vi "PECT - Scan_time gate_counter -XSeries.vi"() -> ()   [LabVIEW 2018]
uses:
  <vilib>/DAQmx/read.llb/DAQmx Read (Counter U32 1Chan 1Samp).vi
  <vilib>/DAQmx/read.llb/DAQmx Read (Analog 2D DBL NChan NSamp).vi
  <vilib>/Instr/_visa.llb/VISA Configure Serial Port (Instr).vi
  <vilib>/DAQmx/create/channels.llb/DAQmx Create Channel (CI-Count Edges).vi
  <vilib>/DAQmx/create/channels.llb/DAQmx Create Channel (AI-Voltage-Basic).vi
  <vilib>/DAQmx/configure/timing.llb/DAQmx Timing (Sample Clock).vi
  <vilib>/DAQmx/configure/trigger.llb/DAQmx Start Trigger (Digital Edge).vi
  <vilib>/DAQmx/miscellaneous.llb/DAQmx Fill In Error Info.vi
  <resource>/objmgr/daqmx.rc
  <vilib>/Platform/NI_3dgraph.lvlib
panel:
  in  "Tab Control 3":enum32{"Control", "Data Processing"}(tab)
  in  "Backdata online":bool caption="Scan"
  in  "Offset":bool
  in  "Open csv":bool
  in  "Scan":bool
  in  "Save Scan mode":bool caption="Save Process"
  in  "Gate 1":dbl=3.0
  in  "Gate 2":dbl=25.0
  in  "Stop Scan":bool
  in  "Right":bool
  in  "Left":bool
  in  "Front":bool
  in  "Back":bool
  in  "Home X":bool
  in  "Home Y":bool
  in  "Stop 3":bool
  in  "Emergency Stop":bool
  in  "Move Distance":dbl=5.0
  in  "Open tdms":bool
  in  "Pulse frequency":dbl=1000.0 format="%0.2p"
  in  "Pulser Cycles":i32=10
  in  "Sensor No.":i32
  in  "Graph":bool
  in  "Sensor Index":dbl[](array[numeric])=[5.0, 10.0, 12.0, 15.0, 19.0]
  in  "Inverse":bool caption="Scan"
  in  "Trim data":bool caption="Scan"
  in  "X-min":dbl
  in  "X-max":dbl
  in  "Y-min":dbl
  in  "Y-max":dbl
  in  "ViewMode":i32(ring) items=["cwViewXYPlane", "cwViewXZPlane", "cwViewYZPlane", "cwViewUserDefined"]
  in  "Plot style":i32(ring)=5 items=["cwLine"=1, "cwPoint"=2, "cwLinePoint"=3, "cwHiddenLine"=4, "cwSurface"=5, "cwSurfaceLine"=6, "cwSurfaceNormal"=7, "cwContourLine"=8, "cwSurfaceContour"=9]
  in  "Repair Line Col":bool
  in  "Repair Line Row":bool
  in  "Line Col":dbl=167.0
  in  "Line Row":dbl
  in  "low cutoff freq":dbl=40.0 format="%0.2f"
  in  "Filter":bool caption="Scan"
  in  "Backdata":bool caption="Scan"
  in  "Odd":bool caption="Scan"
  in  "DiffY":bool caption="Scan"
  in  "DiffX":bool caption="Scan"
  in  "ColorMapAutoScale":bool=TRUE
  in  "Max":dbl=0.6
  in  "Min":dbl=-0.8
  in  "Abs":bool caption="Scan"
  in  "Backindex":i32
  out "Completed":bool
  out "Start Pos. X":dbl=-55.0 format="%#.4f"
  out "Start. Pos.Y":dbl=-76.83 format="%#.4f"
  in  "Tab Control 2":T1(tab)
  out "Hall sensors signal":dbl[][](graph)
  out "Feature Extraction":dbl(graph)
  in  "3D Surface":refnum<k7>(container)
  out "Record path":path caption="selected path"
  out "Feature extraction scan":dbl[](graph)
  in  "Tab Control":T2(tab)=enum."          DAQ        "
  in  "Step X":dbl=0.5
  out "Move X":bool
  in  "Direction (+)":bool=TRUE
  in  "Step Y":dbl=1.0
  in  "Y-length":dbl=1.0
  in  "X-length":dbl=30.0
  in  "Save Speed":bool
  in  "Cur. Pos Y":dbl=18.8 format="%#.4f"
  in  "Cur. Pos X":dbl=-22.5 format="%#.4f"
  in  "Travel per Pulse (mm)":dbl=0.002
  in  "2 Rate":dbl=0.2
  in  "1 Rate":dbl=0.2
  in  "2 Min":dbl=1.0
  in  "1  Max":dbl=8.0
  in  "2 Max":dbl=8.0
  in  "1 Min":dbl=1.0
  in  "Parity":u16(ring) items=["None", "Odd", "Even", "Mark", "Space"]
  in  "stop bits":u16(ring)=10 items=["1.0"=10, "1.5"=15, "2.0"=20]
  in  "Data bits":u16=8 min=5 max=8 step=1
  in  "Baud Rate":u32=9600
  in  "COM Port":refnum<visa-resource-name>="COM3"
  out "No. X":i32
  out "No. Y":i32
  in  "Counter Terminal":tag="/Dev3/PFI8"
  in  "Counter source":tag="Dev3/ctr0"
  out "No. Data":i32
  out "Motor Pulse Count":u32
  in  "Edge":i32(ring)=10280 items=["Rising"=10280, "Falling"=10171]
  in  "Pulser edge terminal":tag="/Dev3/PFI0"
  out "Sample per Channel AI":dbl
  out "Actual Sample Rate":dbl=500000.0 format="%0.2f"
  in  "Physical Channel":tag="Dev3/ai0:31"
  in  "Min Voltage":dbl=-10.0
  in  "Max Voltage":dbl=10.0
  in  "Terminal Configuration":i32(ring)=10083 items=["default"=-1, "RSE"=10083, "NRSE"=10078, "Differential"=10106, "Pseudodifferential"=12529]
  in  "Sample Rate":dbl=30000.0
  in  "Save Scan mode 2":bool caption="Save Process"
  # "Pulse setting"
  # "Data Processing"
  # "Time gate = %T/2"
  # "Motor control"
  # "Color map"
  # "Process"
  # "Repair line"
  # "Hall Sensors Signal"
  # "Feature Extraction"
  # "COM  Setting"
  # "Speed  Setting"
  # "Scan  Setting"
  # "Pulser"
  # "Motor Trigger"
  # "Sensor  Channel"
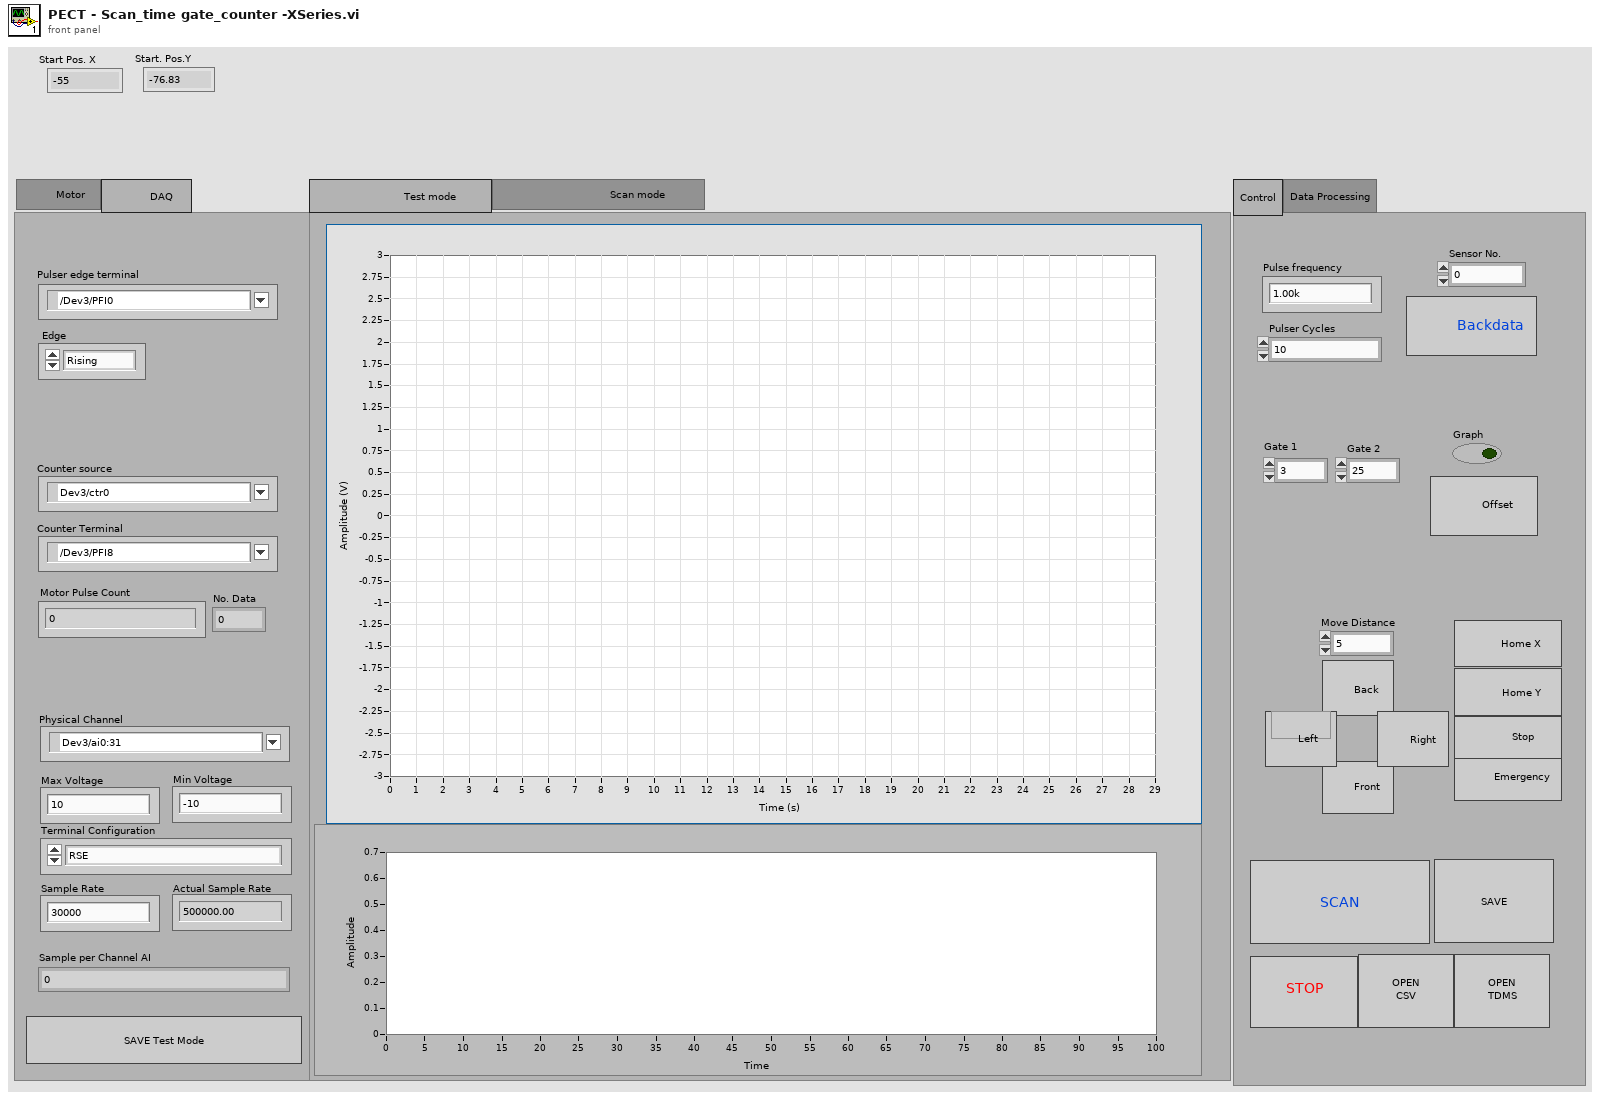
[diagram p1: front panel]
types:
  T1 = enum32{"                    Test mode                   ", "                          Scan mode                      "}
  T2 = enum32{"        Motor      ", "          DAQ        "}
  T3 = enum16{"No Scan", "Move X", "Wait to destination X", "Move Y", "Wait to destinatioin Y"}
  T4 = enum16{"open", "open or create", "create or replace", "create", "open (read-only)"}
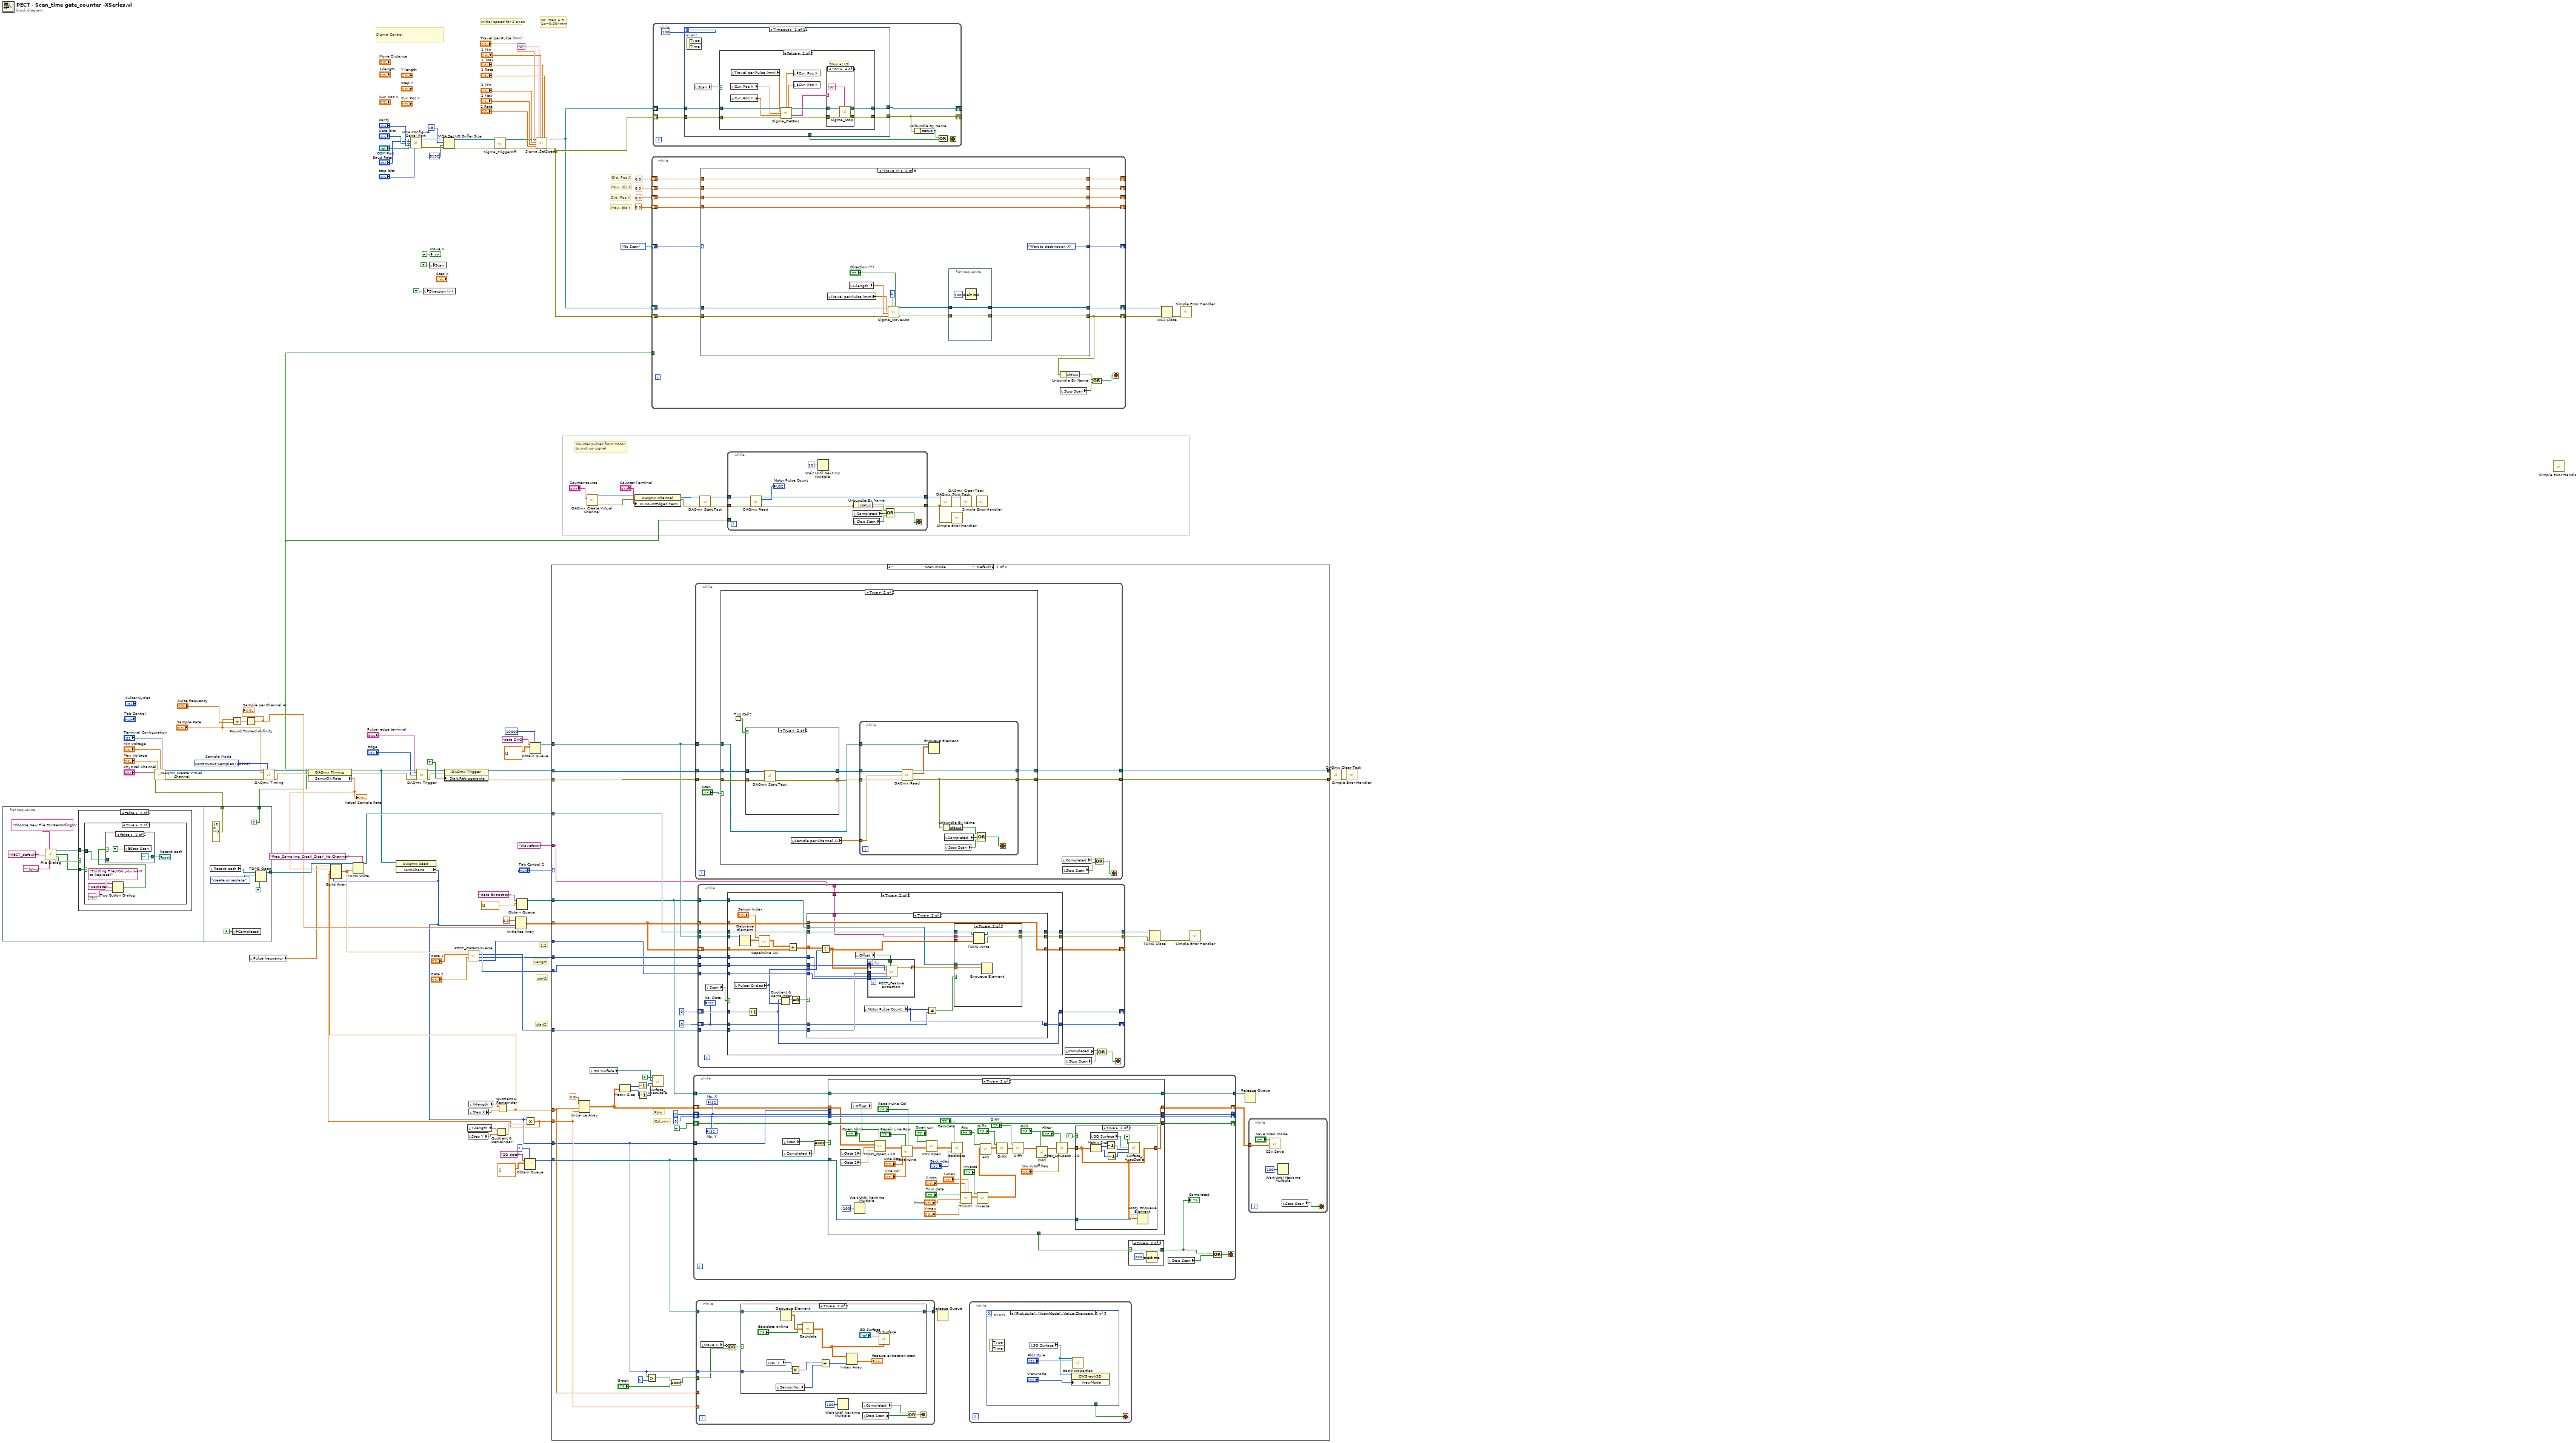
[diagram p0: block diagram]
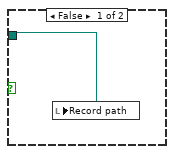
[diagram p2: hidden frame]
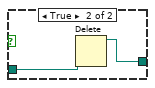
[diagram p3: hidden frame]
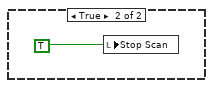
[diagram p4: hidden frame]
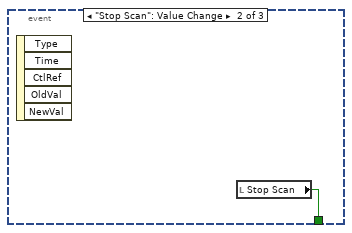
[diagram p5: hidden frame]
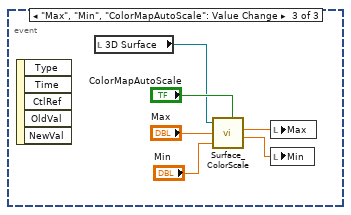
[diagram p6: hidden frame]
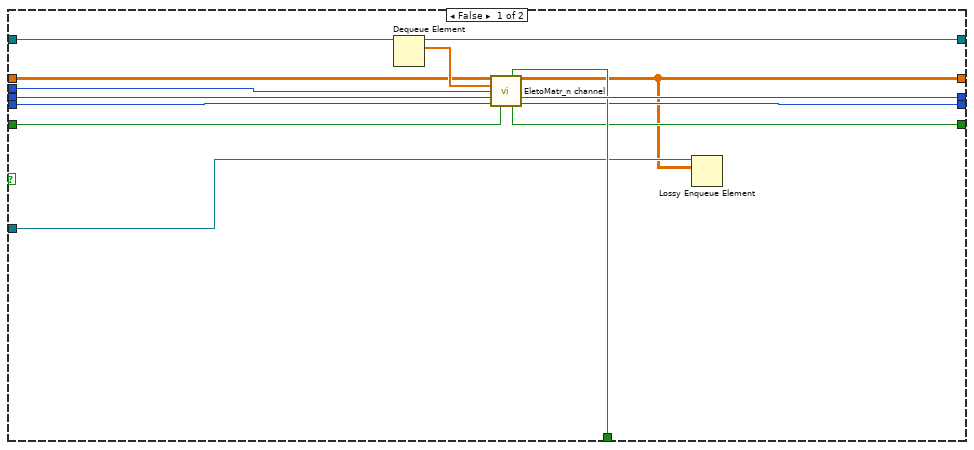
[diagram p9: hidden frame]
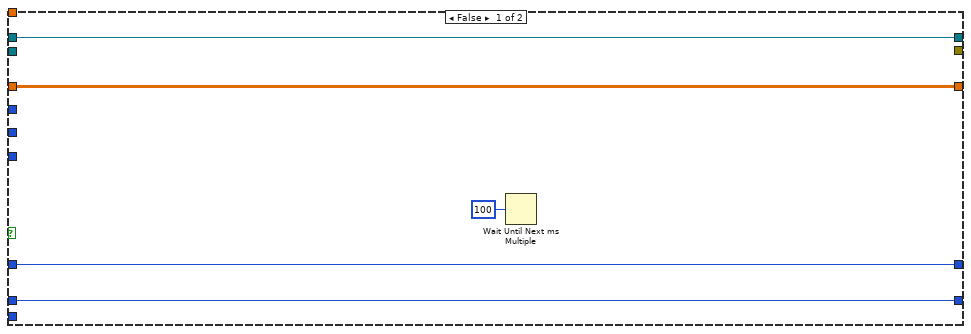
[diagram p13: hidden frame]
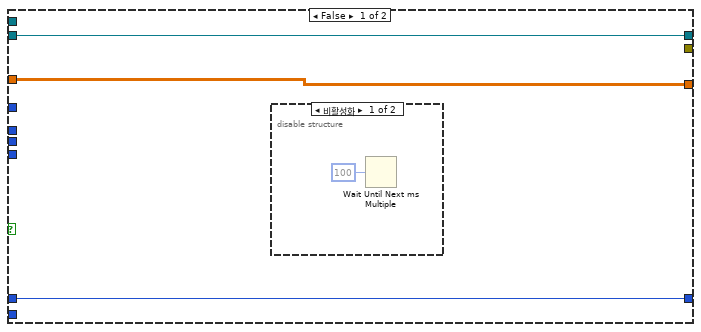
[diagram p14: hidden frame]
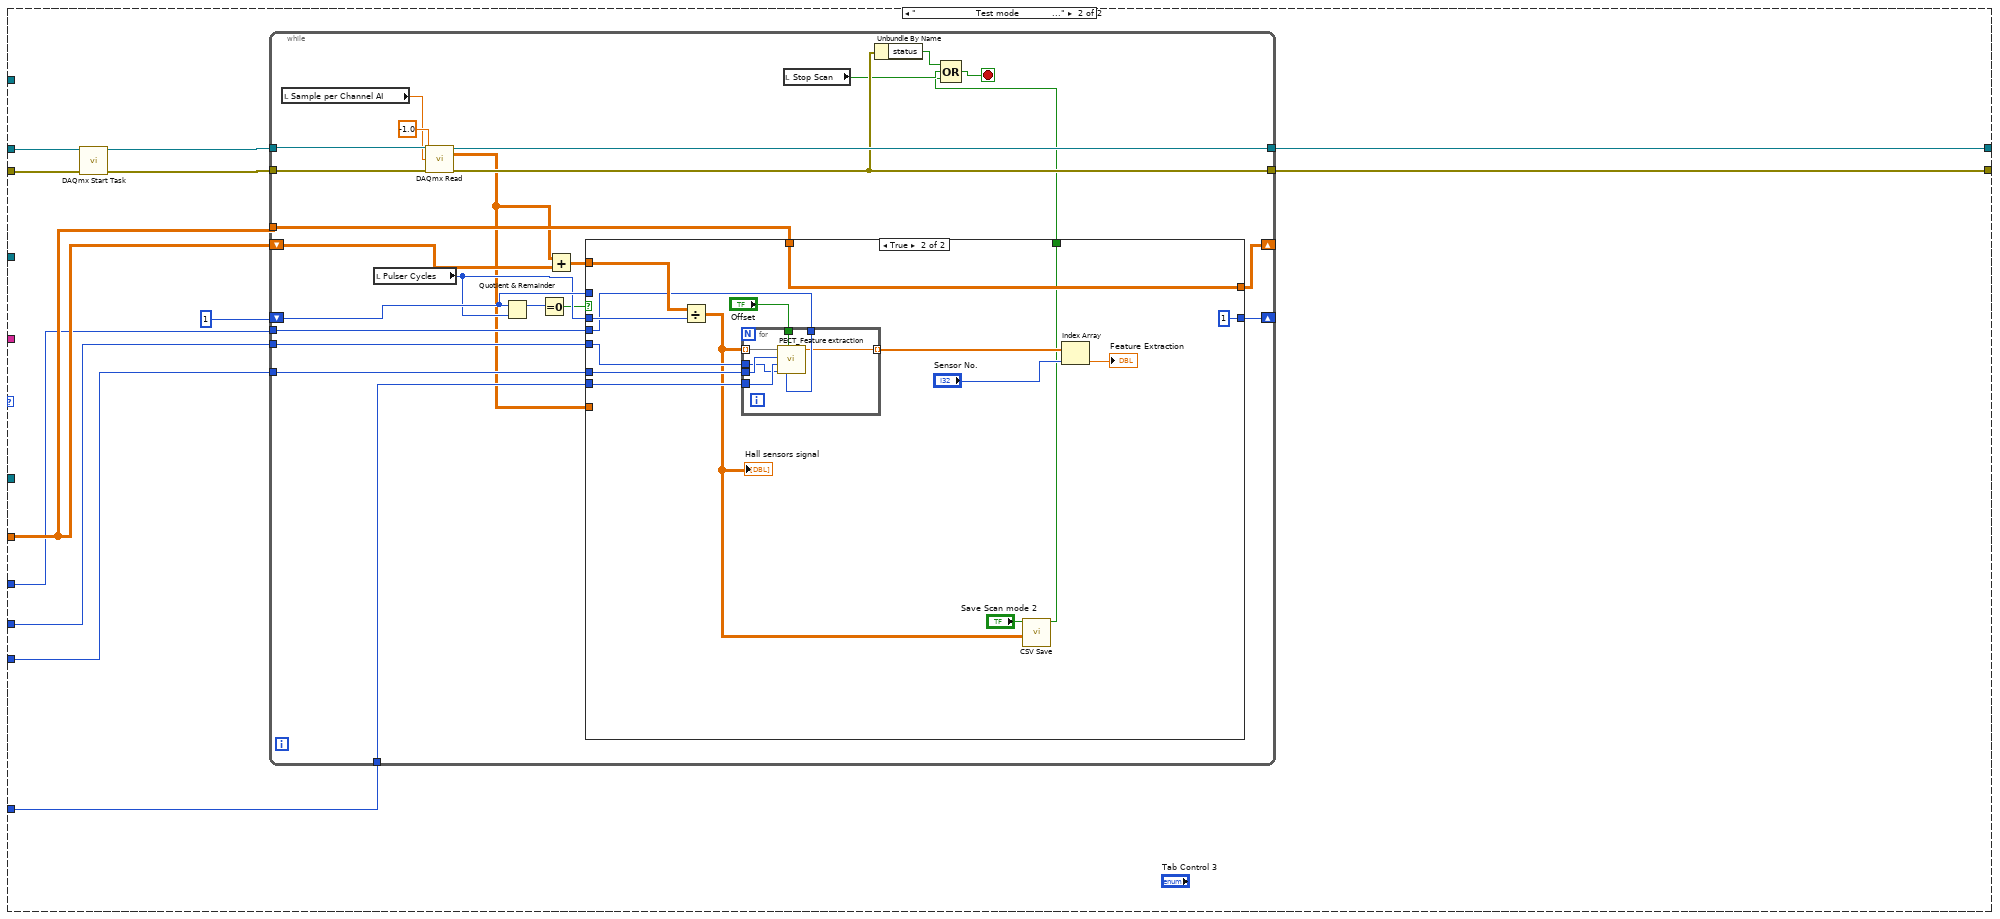
[diagram p17: hidden frame]
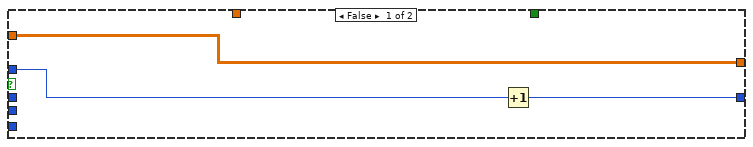
[diagram p18: hidden frame]
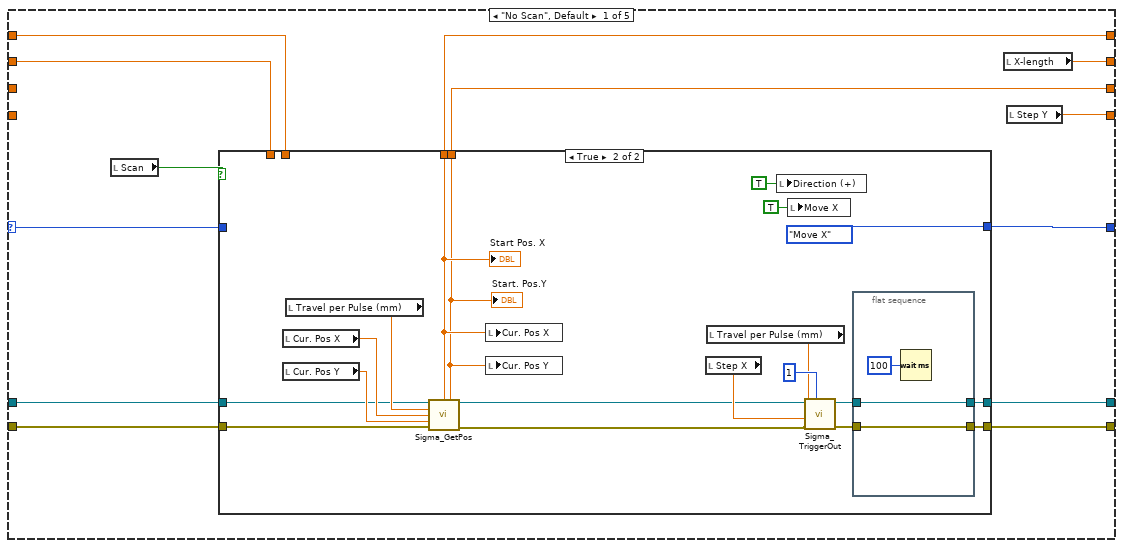
[diagram p19: hidden frame]
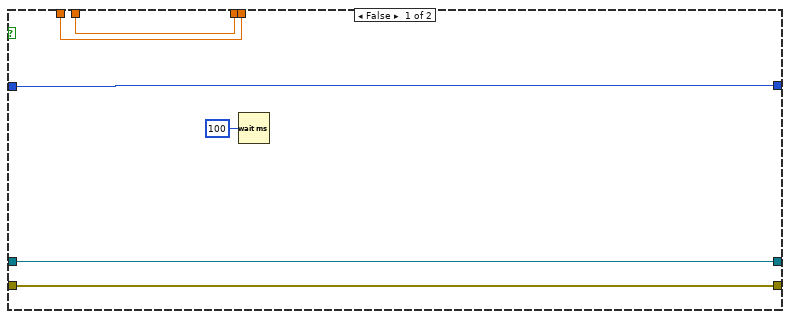
[diagram p20: hidden frame]
diagram:
  w72 = 10123 items=["Finite Samples"=10178, "Continuous Samples"=10123, "Hardware Timed Single Point"=12522]  # Sample Mode
  # "Counter pulses from Motor\nto pick up signal"
  # "1/2"
  # "start1"
  # "start2"
  # "Length"
  # "Mov. dis Y"
  # "Old. Pos Y"
  # "Mov. dis X"
  # "Old. Pos X"
  # "No. step = 5\n1p~0.004mm"
  # "Initial speed for 2 axes"
  # "Sigma Control"
  n1 = flat-sequence {
    tunnel: [w134] -> w57
    tunnel: [TRUE ("disable buffering (T)")] -> w10
    tunnel: [errorcluster {"status"=FALSE, "code"=0, "source"=""} ("error out")] -> w27
    frame #0 {
      n2 = call "File Dialog"("prompt"="Choose New File For Recording\n" ("button label"), "default name"="PECT_default", "pattern (all files)"="*.tdms") -> ("selected path"=w115:path, "exists"=w110:bool, "cancelled"=w111:bool)  [unwired: 9 in, 1 out]
      n3 = case shown="False" w111 {
        tunnel: w115 -> [w116 _]
        tunnel: w110 -> [w117 _]
        frame False {
          n4 = case shown="True" w117 {
            tunnel: w116 -> [w118 w119]
            frame False {
              n5 = local write "Record path"(w118) -> ()
            }
            frame True {
              n6 = Two Button Dialog(message="Existing File\nDo you want to Replace?", 1:"No" ("F button name (\"Cancel\")"), 2:"Replace" ("T button name (\"OK\")")) -> (T button?=w120:bool)
              n7 = case shown="False" w120 {
                tunnel: w119 -> [_ w128]
                tunnel: [path "" ("deleted path") w127] -> w121
                frame False {
                  n8 = local write "Stop Scan"(TRUE ("Exit")) -> ()
                }
                frame True {
                  n9 = Delete(path (use dialog)=w128) -> (deleted path=w127:path)  [unwired: 4 in, 2 out]
                }
              }
              "Record path" <- w121
            }
          }
        }
        frame True {
          n10 = local write "Stop Scan"(TRUE ("Exit")) -> ()
        }
      }
    }
    frame #1 {
      n11 = local read "Record path"() -> (w133:path)
      n12 = local write "Completed"(FALSE ("Completed")) -> ()
      n13 = TDMS Open(6:FALSE ("disable buffering (T)"), 10:T4."create or replace" ("operation"), 11:w133) -> (3:w134:refnum<k34>)  [unwired: 4 in, 1 out]
    }
  }
  n14 = call-poly <vilib>:"DAQmx Create Virtual Channel.vi"("maximum value"="Max Voltage", "minimum value"="Min Voltage", "input terminal configuration"="Terminal Configuration", "physical channels"="Physical Channel", "error in"=w27) -> ("task out"=w81:refnum<k21>, "error out"=w82:errorcluster)  [unwired: 9 in]
  n15 = Divide(x="Sample Rate", y="Pulse frequency") -> (x/y=w59:dbl)
  n16 = Round Toward -Infinity(1:w59) -> (0:w32:dbl)
  "Sample per Channel AI" <- w32
  n17 = local read "Pulse frequency"() -> (w30:dbl)
  n18 = call-poly <vilib>:"DAQmx Timing.vi"("task/channels in"=w81, "sample mode"=w72, "rate"="Sample Rate", "error in"=w82) -> ("task out"=w33:refnum<k21>, "error out"=w83:errorcluster)  [unwired: 10 in]
  n19 = property class="DAQmx Timing"(reference=w33, error in=w83) -> (reference out=w6:refnum<k21>, error out=w3:errorcluster, "SampClk.Rate"=w35:dbl)
  "Actual Sample Rate" <- w35
  n20 = property class="DAQmx Read"(reference=w6) -> ("NumChans"=w26:u32)  [unwired: 1 in, 2 out]
  n21 = call-poly "VISA Configure Serial Port"("VISA resource name"="COM Port", "baud rate (9600)"="Baud Rate", "data bits (8)"="Data bits", "parity (0:none)"="Parity", "stop bits (10: 1 bit)"="stop bits") -> ("VISA resource name out"=w96:refnum<visa-resource-name>, "error out"=w102:errorcluster)  [unwired: 9 in]
  n22 = call-poly <vilib>:"DAQmx Trigger.vi"("task/channels in"=w6, "source"="Pulser edge terminal", "edge"="Edge", "error in"=w3) -> ("task out"=w8:refnum<k21>, "error out"=w7:errorcluster)  [unwired: 10 out]
  n23 = local write "Direction (+)"(TRUE ("Scan")) -> ()
  n24 = local write "Scan"(FALSE ("Scan")) -> ()
  n25 = VISA Set I/O Buffer Size(VISA resource name=w96, mask (16)=48, size (4096)=u32 8192, error in (no error)=w102) -> (VISA resource name out=w44:refnum<visa-resource-name>, error out=w43:errorcluster)
  n26 = property class="DAQmx Trigger"(reference=w8, error in=w7, "Start.Retriggerable"=TRUE) -> (reference out=w5:refnum<k21>, error out=w4:errorcluster)
  n27 = local read "Y-length"() -> (w61:dbl)
  n28 = local read "Step Y"() -> (w62:dbl)
  n29 = local read "X-length"() -> (w64:dbl)
  n30 = local read "Step X"() -> (w63:dbl)
  n31 = call "Sigma_TriggerOff.vi"("error in (no error)"=w43, "VISA resource name"=w44) -> ("error out"=w41:errorcluster, "VISA resource name out"=w42:refnum<visa-resource-name>)  [unwired: 8 in]
  n32 = Quotient & Remainder(x=w61, y=w62) -> (floor(x/y)=w28:dbl)  [unwired: 1 out]
  n33 = Quotient & Remainder(x=w64, y=w63) -> (floor(x/y)=w55:dbl)  [unwired: 1 out]
  n34 = Initialize Array(0.0 ("element"), w26, w32) -> (w69:dbl[][])
  n35 = Obtain Queue(name (unnamed)="data Extraction", element data type=dbl[] [] ("data")) -> (queue out=w66:refnum<queue>)  [unwired: 3 in, 2 out]
  n36 = Obtain Queue(max queue size (-1, unlimited)=2 ("최대 큐 크기(-1,제한없음)"), name (unnamed)="2D data", element data type=dbl[][] [] ("initialized array")) -> (queue out=w37:refnum<queue>)  [unwired: 2 in, 2 out]
  n37 = Multiply(x=w26, y=w28) -> (x*y=w25:dbl)
  n38 = Build Array(w30, w35, w55, w25, w26) -> (w40:dbl[])
  n39 = TDMS Write(0:w57, 5:"Freq_Sampling_SizeX_SizeY_No.Channel" ("group name in (Untitled)"), 9:w40) -> (4:w56:refnum<k34>)  [unwired: 3 in, 3 out]
  n40 = call "PECT_GateConverse.vi"("Gate 2"="Gate 2", "Gate 1"="Gate 1", "Freq_Sampling_SizeX_SizeY"=w40) -> ("Length T/2"=w45:i32, "Length"=w46:i32, "Start 2"=w47:i32, "Start 1"=w48:i32)  [unwired: 4 in, 1 out]
  n41 = Obtain Queue(max queue size (-1, unlimited)=10000, name (unnamed)="data DAQ", element data type=dbl[][] [] ("data")) -> (queue out=w68:refnum<queue>)  [unwired: 2 in, 2 out]
  n42 = call "Sigma_SetSpeed.vi"("VISA resource name"=w42, "Travel per Pulse (0.004mm)"="Travel per Pulse (mm)", "Min (1mm) 2"="2 Min", "Max (2mm) 2"="2 Max", "Rate (1mm) 2"="2 Rate", "error in (no error)"=w41, "Axis (1)"="W", "Min (1mm)"="1 Min", "Max (2mm)"="1  Max", "Rate (1mm)"="1 Rate") -> ("VISA resource name out"=w108:refnum<visa-resource-name>, "error out"=w109:errorcluster)  [unwired: 8 in]
  n43 = case shown="\"                          Scan mode                      \", Default" "Tab Control 2" {
    tunnel: w5 -> [w176 w430]
    tunnel: [w175 w438] -> w75
    tunnel: [w174 w437] -> w74
    tunnel: w69 -> [w171 w436]
    tunnel: w4 -> [w173 w429]
    tunnel: w45 -> [w172 w435]
    tunnel: w68 -> [w170 _]
    tunnel: w66 -> [w150 _]
    tunnel: w55 -> [w145 _]
    tunnel: w25 -> [w146 _]
    tunnel: w46 -> [w158 w433]
    tunnel: w48 -> [w157 w432]
    tunnel: w47 -> [w156 w431]
    tunnel: w56 -> [w155 _]
    tunnel: "Waveform" ("group name in (Untitled)") -> [w152 _]
    tunnel: w37 -> [w147 _]
    tunnel: w26 -> [w141 _]
    frame "                          Scan mode                      ", Default {
      # "Column"
      # "Row"
      n44 = Initialize Array(0.0 ("element"), w145, w146) -> (w142:dbl[][])
      n45 = local read "3D Surface"() -> (w159:refnum<k7>)
      n46 = Matrix Size(0:w142) -> (1:w164:i32, 2:w165:i32)
      n47 = Decrement(x=w164) -> (x-1=w168:i32)
      n48 = Decrement(x=w165) -> (x-1=w167:i32)
      n49 = Greater?(x=w141, y=u32 1) -> (0:w139:bool)
      n50 = call "Surface_AxesScale.vi"("Y-axis Max"=w167, "X-axis max"=w168, "3D Surface"=w159, "Auto Scale"=FALSE) -> ()  [unwired: 8 in]
      n51 = Compound Arithmetic op=AND(w139, "Graph") -> (w137:bool)
      n52 = while {
        shift-right: [w231] -> _
        shift-left: 0 -> [w233]
        shift-right: [w230] -> _
        shift-left: 0 -> [w232]
        tunnel: w150 -> [w229]
        shift-right: [w221] -> w143
        shift-left: w142 -> [w228]
        shift-right: [w224] -> _
        shift-left: TRUE ("Output Direction") -> [w225]
        tunnel: w147 -> [w223]
        tunnel: [w222] -> w148
        tunnel: w141 -> [w217]
        stop <- w226 stop-if-true
        n53 = local read "Scan"() -> (w220:bool)
        n54 = local read "Completed"() -> (w219:bool)
        n55 = Compound Arithmetic op=AND(invert w220, invert w219) -> (w218:bool)
        n56 = case shown="True" w218 {
          tunnel: w233 -> [w250 w293]
          tunnel: w232 -> [w249 w292]
          tunnel: [w248 w293] -> w231
          tunnel: [w243 w292] -> w230
          tunnel: w229 -> [w247 w284]
          tunnel: w228 -> [w238 w289]
          tunnel: [w241 w271] -> w221
          tunnel: [w246 _] -> w216
          tunnel: w225 -> [w245 w291]
          tunnel: [w244 w291] -> w224
          tunnel: w223 -> [w242 w273]
          tunnel: [w237 w284] -> w222
          tunnel: w217 -> [w239 _]
          frame False {
            n57 = Dequeue Element(queue=w247) -> (queue out=w237:refnum<queue>, element=w240:dbl[])  [unwired: 2 in, 2 out]
            n58 = call "EletoMatr_n channel.vi"("Input Array X"=w238, "Input data"=w240, "No. channels"=w239, "In Row"=w250, "In Column"=w249, "Input Direction"=w245) -> ("Completed"=w246:bool, "Out Array X"=w241:dbl[][], "Out Row"=w248:i32, "Output Direction"=w244:bool, "Out Column"=w243:i32)  [unwired: 5 in]
            n59 = Lossy Enqueue Element(queue=w242, element=w241) -> ()  [unwired: 1 in, 4 out]
          }
          frame True {
            n60 = local read "Gate 1"() -> (w288:dbl)
            n61 = local read "Gate 2"() -> (w287:dbl)
            n62 = local read "Offset"() -> (w278:bool)
            n63 = Wait Until Next ms Multiple(millisecond multiple=u32 100 ("ms 배수")) -> ()  [unwired: 1 out]
            n64 = call "TDMS_Open - 1D.vi"("Offset"=w278, "Gate 2"=w287, "Gate 1"=w288, "Input 2D"=w289, "Open"="Open tdms") -> ("Output 2D"=w265:dbl[][])  [unwired: 5 in, 1 out]
            n65 = call "RepairLine.vi"("Repair Line Col"="Repair Line Col", "Repair Line Row"="Repair Line Row", "Line Col"="Line Col", "Line Row"="Line Row", "Array In"=w265) -> ("Array Repaired"=w264:dbl[][])  [unwired: 6 in]
            n66 = call "CSV Open.vi"("2D Array In"=w264, "Open"="Open csv") -> ("2D Array Out"=w272:dbl[][])  [unwired: 9 in]
            n67 = call "Backdata.vi"("Backindex"="Backindex", "Array in"=w272, "Backdata"="Backdata") -> ("Array out"=w259:dbl[][])
            n68 = call "TrimXY.vi"("X-max"="Y-max", "X-min"="Y-min", "Y-max"="X-max", "Y-min"="X-min", "Array In"=w259, "Trim data"="Trim data") -> ("Array Trim Out"=w253:dbl[][])  [unwired: 5 in]
            n69 = call "Inverse.vi"(10:"Inverse"=w253, 11:"Inverse"="Inverse") -> ("Array out"=w251:dbl[][])  [unwired: 9 in]
            n70 = call "Abs.vi"("Input"=w251, "Abs"="Abs") -> ("Array out"=w277:dbl[][])  [unwired: 9 in]
            n71 = call "DiffX.vi"("Array in"=w277, "DiffX"="DiffX") -> ("Array out"=w282:dbl[][])  [unwired: 1 in]
            n72 = call "DiffY.vi"("Array in"=w282, "DiffY"="DiffY") -> ("Array out"=w280:dbl[][])  [unwired: 1 in]
            n73 = call "Odd.vi"("Odd"="Odd", "Array In"=w280) -> ("Array Out"=w269:dbl[][])  [unwired: 9 in]
            n74 = call "Filter_Lowpass - 2D.vi"("Filter"="Filter", "Input 2D"=w269, "low cutoff freq: fl"="low cutoff freq") -> ("Output"=w268:dbl[][])  [unwired: 6 in]
            n75 = case shown="True" TRUE {
              tunnel: w268 -> [w294 w295]
              tunnel: [w294 w295] -> w271
              tunnel: w273 -> [_ w296]
              frame False {
              }
              frame True {
                n76 = local read "3D Surface"() -> (w300:refnum<k7>)
                n77 = Matrix Size(0:w295) -> (1:w301:i32, 2:w298:i32)
                n78 = Decrement(x=w301) -> (x-1=w299:i32)
                n79 = Decrement(x=w298) -> (x-1=w297:i32)
                n80 = call "Surface_AxesScale.vi"("Y-axis Max"=w297, "X-axis max"=w299, "3D Surface"=w300, "Auto Scale"=FALSE) -> ()  [unwired: 8 in]
                n81 = Lossy Enqueue Element(queue=w296, element=w295) -> ()  [unwired: 1 in, 4 out]
              }
            }
          }
        }
        n82 = case shown="True" w216 {
          selector: w216 -> [w234 w235]
          tunnel: [w234 w235] -> w215
          frame False {
          }
          frame True {
            n83 = Wait (ms)(milliseconds to wait=u32 200) -> ()  [unwired: 1 out]
          }
        }
        "Completed" <- w215
        n84 = local read "Stop Scan"() -> (w227:bool)
        n85 = Compound Arithmetic op=OR(w215, w227) -> (w226:bool)
        "No. Y" <- w232
        "No. X" <- w233
      }
      n86 = while {
        tunnel: w176 -> [w311]
        tunnel: [w310] -> w175
        tunnel: [w309] -> w174
        tunnel: w173 -> [w308]
        tunnel: w170 -> [w307]
        stop <- w303 stop-if-true
        n87 = case shown="True" "Scan" {
          tunnel: w311 -> [w313 w320]
          tunnel: [w313 w322] -> w310
          tunnel: [w312 w321] -> w309
          tunnel: w308 -> [w312 w319]
          tunnel: w307 -> [_ w316]
          frame False {
          }
          frame True {
            n88 = First Call?() -> (First Call?: T/F=w315:bool)
            n89 = case shown="True" w315 {
              tunnel: w320 -> [w324 w328]
              tunnel: w319 -> [w323 w327]
              tunnel: [w324 w326] -> w318
              tunnel: [w323 w325] -> w317
              frame False {
              }
              frame True {
                n90 = call <vilib>:"DAQmx Start Task.vi"("task/channels in"=w328, "error in"=w327) -> ("task out"=w326:refnum<k21>, "error out"=w325:errorcluster)  [unwired: 12 in]
              }
            }
            n91 = local read "Sample per Channel AI"() -> (w314:dbl)
            n92 = while {
              tunnel: [w339] -> w322
              tunnel: [w338] -> w321
              tunnel: w316 -> [w337]
              tunnel: w318 -> [w332]
              tunnel: w317 -> [w331]
              tunnel: w314 -> [w329]
              stop <- w333 stop-if-true
              n93 = call-poly <vilib>:"DAQmx Read.vi"("task/channels in"=w332, "number of samples per channel"=w329, "error in"=w331) -> ("task out"=w339:refnum<k21>, "data"=w330:dbl[][], "error out"=w338:errorcluster)  [unwired: 10 in]
              n94 = Enqueue Element(queue=w337, element=w330) -> ()  [unwired: 2 in, 3 out]
              n95 = Unbundle By Name(w338) -> ("status"=w334:bool)
              n96 = local read "Completed"() -> (w336:bool)
              n97 = local read "Stop Scan"() -> (w335:bool)
              n98 = Compound Arithmetic op=OR(w334, w336, w335) -> (w333:bool)
            }
          }
        }
        n99 = local read "Completed"() -> (w304:bool)
        n100 = local read "Stop Scan"() -> (w305:bool)
        n101 = Compound Arithmetic op=OR(w304, w305) -> (w303:bool)
      }
      n102 = while {
        tunnel: w147 -> [w195]
        tunnel: w146 -> [_]
        tunnel: w145 -> [_]
        tunnel: [w198] -> w144
        tunnel: w141 -> [w197]
        tunnel: w137 -> [w193]
        stop <- w199 stop-if-true
        n103 = local read "Move X"() -> (w194:bool)
        n104 = Compound Arithmetic op=OR(invert w194, w193) -> (w192:bool)
        n105 = case shown="True" w192 {
          tunnel: [w202 w212] -> w198
          tunnel: w197 -> [_ w210]
          tunnel: w195 -> [w202 w206]
          frame False {
          }
          frame True {
            n106 = local read "No. Y"() -> (w211:i32)
            n107 = local read "Sensor No."() -> (w208:i32)
            n108 = Dequeue Element(queue=w206) -> (queue out=w212:refnum<queue>, element=w205:dbl[][])  [unwired: 2 in, 2 out]
            n109 = Multiply(x=w211, y=w210) -> (x*y=w209:u32)
            n110 = call "Backdata.vi"("Array in"=w205, "Backdata"="Backdata online") -> ("Array out"=w204:dbl[][])  [unwired: 1 in]
            n111 = Add(x=w209, y=w208) -> (x+y=w207:u32)
            n112 = Index Array(array=w204, index (col)=w207) -> (element=→"Feature extraction scan":dbl[])  [unwired: 1 in]
            n113 = call <vilib>:"3D Surface.vi"("z matrix"=w204, "3D graph"="3D Surface") -> ()  [unwired: 8 in, 2 out]
          }
        }
        n114 = Wait Until Next ms Multiple(millisecond multiple=u32 100 ("ms 배수")) -> ()  [unwired: 1 out]
        n115 = local read "Completed"() -> (w196:bool)
        n116 = local read "Stop Scan"() -> (w200:bool)
        n117 = Compound Arithmetic op=OR(w196, w200) -> (w199:bool)
      }
      n118 = while {
        shift-right: [w356] -> _
        shift-left: w171 -> [w360]
        tunnel: w171 -> [w359]
        tunnel: w172 -> [w358]
        tunnel: w170 -> [w357]
        tunnel: w150 -> [w355]
        shift-right: [w352] -> _
        shift-left: 0 -> [w353]
        tunnel: w158 -> [w351]
        tunnel: w157 -> [w350]
        tunnel: w156 -> [w349]
        tunnel: w155 -> [w348]
        tunnel: [w347] -> w154
        tunnel: [w346] -> w153
        tunnel: w152 -> [w345]
        shift-right: [w344] -> _
        shift-left: 0 -> [w340]
        stop <- w341 stop-if-true
        n119 = local read "Scan"() -> (w354:bool)
        n120 = case shown="True" w354 {
          tunnel: w360 -> [w365 w381]
          tunnel: w359 -> [_ w386]
          tunnel: w358 -> [_ w385]
          tunnel: w357 -> [_ w384]
          tunnel: [w365 w383] -> w356
          tunnel: w355 -> [_ w382]
          tunnel: w353 -> [w364 w379]
          tunnel: [w364 w378] -> w352
          tunnel: w351 -> [_ w377]
          tunnel: w350 -> [_ w376]
          tunnel: w349 -> [_ w375]
          tunnel: w348 -> [w362 w374]
          tunnel: [w362 w373] -> w347
          tunnel: [_ w372] -> w346
          tunnel: w345 -> [_ w371]
          tunnel: w340 -> [w361 w370]
          tunnel: [w361 w369] -> w344
          frame False {
            n121 = Wait Until Next ms Multiple(millisecond multiple=u32 100 ("ms 배수")) -> ()  [unwired: 1 out]
          }
          frame True {
            n122 = local read "Pulser Cycles"() -> (w380:i32)
            n123 = Dequeue Element(queue=w384) -> (element=w368:dbl[][])  [unwired: 2 in, 3 out]
            n124 = Increment(x=w379) -> (x+1=w378:i32)
            n125 = call "RepairLine 2D.vi"("Array in"=w368, "Sensor Index"="Sensor Index") -> ("Array Out"=w366:dbl[][])  [unwired: 9 in]
            n126 = Quotient & Remainder(x=w378, y=w380) -> (x-y*floor(x/y)=w387:i32)  [unwired: 1 out]
            n127 = Add(x=w366, y=w381) -> (x+y=w389:dbl[][])
            n128 = Equal To 0?(x=w387) -> (x = 0?=w388:bool)
            n129 = case shown="True" w388 {
              tunnel: w380 -> [_ w410]
              tunnel: w389 -> [w392 w408]
              tunnel: [w392 w411] -> w383
              tunnel: w386 -> [_ w411]
              tunnel: w385 -> [_ w404]
              tunnel: w382 -> [_ w409]
              tunnel: w377 -> [_ w405]
              tunnel: w376 -> [_ w407]
              tunnel: w375 -> [_ w406]
              tunnel: w374 -> [w391 w400]
              tunnel: [w391 w397] -> w373
              tunnel: [_ w396] -> w372
              tunnel: w371 -> [_ w399]
              tunnel: w370 -> [w390 w401]
              tunnel: [w390 w395] -> w369
              frame False {
                n130 = disable-structure shown="비활성화" {
                  frame Disabled {
                    n131 = Wait Until Next ms Multiple(millisecond multiple=u32 100 ("ms 배수")) -> ()  [unwired: 1 out]
                  }
                  frame Enabled {
                  }
                }
              }
              frame True {
                n132 = Divide(x=w408, y=w410) -> (x/y=w398:dbl[][])
                n133 = local read "Offset"() -> (w403:bool)
                n134 = local read "Motor Pulse Count"() -> (w395:u32)
                n135 = for {
                  tunnel: w407 -> [w418]
                  tunnel: w406 -> [w417]
                  tunnel: w405 -> [w416]
                  tunnel: w404 -> [w415]
                  tunnel: w403 -> [w414]
                  tunnel: [w413] -> w402 mode=indexing
                  tunnel: w398 -> [w412] mode=indexing
                  n136 = call "PECT_Feature extraction.vi"("Length T/2"=w415, "Offset"=w414, "Length"=w416, "Start 2"=w417, "Start 1"=w418, "Pulse signal in"=w412) -> ("Feature extraction out"=w413:dbl)  [unwired: 5 in]
                }
                n137 = Not Equal?(x=w395, y=w401) -> (x != y?=w394:bool)
                n138 = case shown="True" w394 {
                  tunnel: w409 -> [_ w426]
                  tunnel: w402 -> [_ w425]
                  tunnel: w400 -> [w419 w424]
                  tunnel: w399 -> [_ w423]
                  tunnel: w398 -> [_ w422]
                  tunnel: [w419 w421] -> w397
                  tunnel: [_ w420] -> w396
                  frame False {
                  }
                  frame True {
                    n139 = TDMS Write(0:w424, 5:w423, 9:w422) -> (4:w421:refnum<k34>, 15:w420:errorcluster)  [unwired: 3 in, 2 out]
                    n140 = Enqueue Element(queue=w426, element=w425) -> ()  [unwired: 2 in, 3 out]
                  }
                }
              }
            }
          }
        }
        n141 = local read "Completed"() -> (w343:bool)
        n142 = local read "Stop Scan"() -> (w342:bool)
        n143 = Compound Arithmetic op=OR(w343, w342) -> (w341:bool)
        "No. Data" <- w340
      }
      n144 = Release Queue(queue=w144) -> ()  [unwired: 2 in, 3 out]
      n145 = while {
        stop <- w181 stop-if-true
        n146 = event shown="[0] \"Plot style\", \"ViewMode\": Value Change" {
          selector: _ -> [_ _ _]
          dyn-events: _ -> [_ _ _]
          timeout: _ -> [_ _ _]
          tunnel: [_ w185 _] -> w181
          event "Plot style", "ViewMode": Value Change {
            n147 = event-data() -> ()  [unwired: 1 in, 2 out]
            n148 = local read "3D Surface"() -> (w184:refnum<k7>)
            n149 = property class="CWGraph3D"(reference=w184, "ViewMode"="ViewMode") -> ()  [unwired: 1 in, 2 out]
            n150 = call <vilib>:"Basic Properties.vi"("3D graph"=w184, "plot style"="Plot style") -> ()  [unwired: 12 in, 2 out]
          }
          event "Stop Scan": Value Change {
            n151 = event-data() -> ()  [unwired: 1 in, 5 out]
            n152 = local read "Stop Scan"() -> (w185:bool)
          }
          event "Max", "Min", "ColorMapAutoScale": Value Change {
            n153 = event-data() -> ()  [unwired: 1 in, 5 out]
            n154 = local read "3D Surface"() -> (w186:refnum<k7>)
            n155 = call "Surface_ColorScale.vi"("ColorMapAutoScale"="ColorMapAutoScale", "Min"="Min", "Max"="Max", "3D Surface_"=w186) -> ("Min 2"=w190:dbl, "Max 2"=w189:dbl)  [unwired: 1 in, 2 out]
            n156 = local write "Max"(w189) -> ()
            n157 = local write "Min"(w190) -> ()
          }
        }
      }
      n158 = TDMS Close(8:w153, 11:w154) -> (0:w151:errorcluster)  [unwired: 1 out]
      n159 = call <vilib>:"Simple Error Handler.vi"("error in (no error)"=w151) -> ()  [unwired: 2 in, 7 out]
      n160 = Release Queue(queue=w148) -> ()  [unwired: 2 in, 3 out]
      n161 = while {
        tunnel: w143 -> [w179]
        stop <- w178 stop-if-true
        n162 = call "CSV Save.vi"("Array"=w179, "Save Button"="Save Scan mode") -> ()  [unwired: 9 in, 1 out]
        n163 = Wait Until Next ms Multiple(millisecond multiple=u32 100 ("ms 배수")) -> ()  [unwired: 1 out]
        n164 = local read "Stop Scan"() -> (w178:bool)
      }
    }
    frame "                    Test mode                   " {
      n165 = call <vilib>:"DAQmx Start Task.vi"("task/channels in"=w430, "error in"=w429) -> ("task out"=w428:refnum<k21>, "error out"=w427:errorcluster)  [unwired: 12 in]
      n166 = while {
        tunnel: w428 -> [w446]
        tunnel: w427 -> [w445]
        tunnel: [w461] -> w437
        tunnel: [w462] -> w438
        shift-right: [w458] -> _
        shift-left: w436 -> [w459]
        tunnel: w436 -> [w457]
        tunnel: w435 -> [w455]
        shift-right: [w453] -> _
        shift-left: 1 ("Average") -> [w452]
        tunnel: w433 -> [w450]
        tunnel: w432 -> [w449]
        tunnel: w431 -> [w448]
        stop <- w439 stop-if-true
        n167 = local read "Sample per Channel AI"() -> (w444:dbl)
        n168 = local read "Pulser Cycles"() -> (w451:i32)
        n169 = call-poly <vilib>:"DAQmx Read.vi"("task/channels in"=w446, "number of samples per channel"=w444, "timeout"=-1.0, "error in"=w445) -> ("task out"=w462:refnum<k21>, "data"=w443:dbl[][], "error out"=w461:errorcluster)  [unwired: 9 in]
        n170 = Quotient & Remainder(x=w452, y=w451) -> (x-y*floor(x/y)=w460:i32)  [unwired: 1 out]
        n171 = Equal To 0?(x=w460) -> (x = 0?=w447:bool)
        n172 = Add(x=w443, y=w459) -> (x+y=w456:dbl[][])
        n173 = case shown="True" w447 {
          tunnel: w451 -> [_ w478]
          tunnel: w443 -> [_ _]
          tunnel: w456 -> [w465 w480]
          tunnel: [w465 w479] -> w458
          tunnel: w457 -> [_ w479]
          tunnel: w455 -> [_ w472]
          tunnel: [w463 1 ("Average")] -> w453
          tunnel: w452 -> [w464 _]
          tunnel: w450 -> [_ w474]
          tunnel: w449 -> [_ w476]
          tunnel: w448 -> [_ w475]
          tunnel: [_ w466] -> w440
          frame False {
            n174 = Increment(x=w464) -> (x+1=w463:i32)
          }
          frame True {
            n175 = Divide(x=w480, y=w478) -> (x/y=w467:dbl[][])
            "Hall sensors signal" <- w467
            n176 = for {
              tunnel: w467 -> [w487] mode=indexing
              tunnel: w476 -> [w486]
              tunnel: w475 -> [w485]
              tunnel: w474 -> [w484]
              tunnel: "Offset" -> [w483]
              tunnel: w472 -> [w482]
              tunnel: [w481] -> w471 mode=indexing
              n177 = call "PECT_Feature extraction.vi"("Length T/2"=w482, "Offset"=w483, "Length"=w484, "Start 2"=w485, "Start 1"=w486, "Pulse signal in"=w487) -> ("Feature extraction out"=w481:dbl)  [unwired: 5 in]
            }
            n178 = call "CSV Save.vi"("Array"=w467, "Save Button"="Save Scan mode 2") -> ("Save Status"=w466:bool)  [unwired: 9 in]
            n179 = Index Array(array=w471, index="Sensor No.") -> (element=→"Feature Extraction":dbl)
          }
        }
        n180 = local read "Stop Scan"() -> (w441:bool)
        n181 = Unbundle By Name(w461) -> ("status"=w442:bool)
        n182 = Compound Arithmetic op=OR(w442, w441, w440) -> (w439:bool)
      }
    }
  }
  n183 = call-poly <vilib>:"DAQmx Create Virtual Channel.vi"("counter"="Counter source") -> ("task out"=w18:refnum<k21>, "error out"=w20:errorcluster)  [unwired: 13 in]
  n184 = property class="DAQmx Channel"(reference=w18, error in=w20, "CI.CountEdges.Term"="Counter Terminal") -> (reference out=w13:refnum<k21>, error out=w14:errorcluster)
  n185 = while {
    shift-right: [w503] -> _
    shift-left: T3."No Scan" -> [w504]
    shift-right: [w499] -> _
    shift-left: 0.0 ("Current  Position (mm)") -> [w498]
    shift-right: [w497] -> _
    shift-left: 0.0 ("Current  Position (mm)") -> [w496]
    shift-right: [w495] -> _
    shift-left: 0.0 ("Current  Position (mm)") -> [w494]
    shift-right: [w493] -> _
    shift-left: 0.0 ("Current  Position (mm)") -> [w492]
    shift-right: [w500] -> w52
    shift-left: w108 -> [w502]
    shift-right: [w490] -> w53
    shift-left: w109 -> [w501]
    tunnel: w10 -> [_]
    stop <- w488 stop-if-true
    n186 = case shown="\"Move X\"" w504 {
      selector: w504 -> [w515 _ _ _ _]
      tunnel: [w516 T3."Wait to destination X" w580 w597 w653] -> w503
      tunnel: w502 -> [w510 w549 w574 w602 w644]
      tunnel: w501 -> [w509 w548 w573 w601 w643]
      tunnel: [w512 w551 w579 w599 w650] -> w500
      tunnel: [w511 w550 w578 w598 w649] -> w490
      tunnel: [w508 w556 w577 w616 w656] -> w499
      tunnel: w498 -> [w506 w556 w565 w616 w656]
      tunnel: [w514 w555 w582 w615 w655] -> w497
      tunnel: w496 -> [w505 w555 w582 w615 w655]
      tunnel: [w507 w554 w575 w600 w652] -> w495
      tunnel: w494 -> [_ w554 w575 w600 w638]
      tunnel: [w513 w553 w583 w614 w651] -> w493
      tunnel: w492 -> [_ w553 w583 w614 w651]
      frame "No Scan", Default {
        n187 = local read "Scan"() -> (w517:bool)
        n188 = case shown="True" w517 {
          tunnel: [w523 T3."Move X"] -> w516
          tunnel: w515 -> [w523 _]
          tunnel: w510 -> [w522 w529]
          tunnel: w509 -> [w521 w528]
          tunnel: [w522 w534] -> w512
          tunnel: [w521 w533] -> w511
          tunnel: [w520 w525] -> w508
          tunnel: [w519 w524] -> w507
          tunnel: w506 -> [w520 _]
          tunnel: w505 -> [w519 _]
          frame False {
            n189 = Wait (ms)(milliseconds to wait=u32 100) -> ()  [unwired: 1 out]
          }
          frame True {
            n190 = local read "Cur. Pos X"() -> (w531:dbl)
            n191 = local read "Cur. Pos Y"() -> (w532:dbl)
            n192 = local read "Travel per Pulse (mm)"() -> (w530:dbl)
            n193 = call "Sigma_GetPos.vi"("VISA resource name"=w529, "Travel per Pulse (mm)"=w530, "Init Pos X (mm)"=w531, "Init  Pos Y (mm)"=w532, "error in (no error)"=w528) -> ("Pos X (mm)"=w525:dbl, "Pos Y (mm)"=w524:dbl, "VISA resource name out"=w527:refnum<visa-resource-name>, "error out"=w526:errorcluster)  [unwired: 6 in, 1 out]
            "Start Pos. X" <- w525
            "Start. Pos.Y" <- w524
            n194 = local write "Cur. Pos X"(w525) -> ()
            n195 = local write "Cur. Pos Y"(w524) -> ()
            n196 = local read "Step X"() -> (w538:dbl)
            n197 = local read "Travel per Pulse (mm)"() -> (w537:dbl)
            n198 = local write "Direction (+)"(TRUE ("Direction (+)")) -> ()
            n199 = local write "Move X"(TRUE ("Move X")) -> ()
            n200 = call "Sigma_TriggerOut.vi"("Axis(1)"=1, "error in (no error)"=w526, "Trigger distance (mm)"=w538, "Travel per Pulse (mm)"=w537, "VISA resource name"=w527) -> ("error out"=w535:errorcluster, "VISA resource name out"=w536:refnum<visa-resource-name>)  [unwired: 5 in]
            n201 = flat-sequence {
              tunnel: [w545] -> w534
              tunnel: w536 -> [w545]
              tunnel: [w544] -> w533
              tunnel: w535 -> [w544]
              frame #0 {
                n202 = Wait (ms)(milliseconds to wait=u32 100) -> ()  [unwired: 1 out]
              }
            }
          }
        }
        n203 = local read "X-length"() -> (w514:dbl)
        n204 = local read "Step Y"() -> (w513:dbl)
      }
      frame "Move X" {
        n205 = local read "Travel per Pulse (mm)"() -> (w558:dbl)
        n206 = local read "X-length"() -> (w559:dbl)
        n207 = call "Sigma_MoveAbs.vi"("Direction (+)"="Direction (+)", "Axis (1)"=1, "error in (no error)"=w548, "Travel (1mm)"=w559, "Travel per Pulse (0.004mm)"=w558, "VISA resource name"=w549) -> ("error out"=w546:errorcluster, "VISA resource name out"=w547:refnum<visa-resource-name>)  [unwired: 4 in]
        n208 = flat-sequence {
          tunnel: [w563] -> w551
          tunnel: w547 -> [w563]
          tunnel: [w562] -> w550
          tunnel: w546 -> [w562]
          frame #0 {
            n209 = Wait (ms)(milliseconds to wait=u32 100) -> ()  [unwired: 1 out]
          }
        }
      }
      frame "Wait to destination X" {
        n210 = local read "Cur. Pos X"() -> (w570:dbl)
        n211 = local read "Cur. Pos Y"() -> (w569:dbl)
        n212 = local read "Travel per Pulse (mm)"() -> (w576:dbl)
        n213 = call "Sigma_GetPos.vi"("VISA resource name"=w574, "Travel per Pulse (mm)"=w576, "Init Pos X (mm)"=w570, "Init  Pos Y (mm)"=w569, "error in (no error)"=w573) -> ("Pos X (mm)"=w564:dbl, "Pos Y (mm)"=w568:dbl, "VISA resource name out"=w572:refnum<visa-resource-name>, "error out"=w571:errorcluster)  [unwired: 6 in, 1 out]
        n214 = Absolute Value(x=w582) -> (abs(x)=w584:dbl)
        n215 = local write "Cur. Pos X"(w564) -> ()
        n216 = local write "Cur. Pos Y"(w568) -> ()
        n217 = Subtract(x=w564, y=w565) -> (x-y=w586:dbl)
        n218 = Absolute Value(x=w586) -> (abs(x)=w585:dbl)
        n219 = Subtract(x=w585, y=w584) -> (x-y=w567:dbl)
        n220 = call "Convert Double Precision.vi"("Input"=w567) -> ("Output"=w566:dbl)  [unwired: 10 in]
        n221 = Greater Or Equal To 0?(x=w566) -> (x >= 0?=w581:bool)
        n222 = case shown="True" w581 {
          tunnel: [T3."Wait to destination X" T3."Move Y"] -> w580
          tunnel: w572 -> [w589 w593]
          tunnel: w571 -> [w588 w592]
          tunnel: [w589 w593] -> w579
          tunnel: [w588 w592] -> w578
          tunnel: [w587 w594] -> w577
          tunnel: w565 -> [w587 _]
          frame False {
            n223 = disable-structure shown="비활성화" {
              frame Disabled {
                n224 = Wait (ms)(milliseconds to wait=u32 100) -> ()  [unwired: 1 out]
              }
              frame Enabled {
              }
            }
          }
          frame True {
            n225 = local read "Cur. Pos X"() -> (w594:dbl)
            n226 = local write "Move X"(FALSE ("Move X")) -> ()
          }
        }
      }
      frame "Move Y" {
        n227 = local read "Y-length"() -> (w605:dbl)
        n228 = local read "Step Y"() -> (w603:dbl)
        n229 = local read "Start. Pos.Y"() -> (w608:dbl)
        n230 = Subtract(x=w605, y=w603) -> (x-y=w604:dbl)
        n231 = Subtract(x=w608, y=w600) -> (x-y=w613:dbl)
        n232 = Absolute Value(x=w604) -> (abs(x)=w611:dbl)
        n233 = Absolute Value(x=w613) -> (abs(x)=w612:dbl)
        n234 = Subtract(x=w612, y=w611) -> (x-y=w606:dbl)
        n235 = local write "Move X"(FALSE ("Move X")) -> ()
        n236 = call "Convert Double Precision.vi"("Input"=w606) -> ("Output"=w607:dbl)  [unwired: 10 in]
        n237 = Greater Or Equal To 0?(x=w607) -> (x >= 0?=w609:bool)
        n238 = case shown="False" w609 {
          tunnel: [w619 w635] -> w599
          tunnel: [w618 w634] -> w598
          tunnel: w602 -> [w621 w633]
          tunnel: w601 -> [w620 w632]
          tunnel: [T3."Wait to destinatioin Y" T3."No Scan"] -> w597
          frame False {
            n239 = local read "Travel per Pulse (mm)"() -> (w625:dbl)
            n240 = local read "Step Y"() -> (w626:dbl)
            n241 = call "Sigma_MoveAbs.vi"("Direction (+)"=TRUE, "Axis (1)"=2, "error in (no error)"=w620, "Travel (1mm)"=w626, "Travel per Pulse (0.004mm)"=w625, "VISA resource name"=w621) -> ("error out"=w623:errorcluster, "VISA resource name out"=w624:refnum<visa-resource-name>)  [unwired: 4 in]
            n242 = flat-sequence {
              tunnel: [w630] -> w619
              tunnel: w624 -> [w630]
              tunnel: [w629] -> w618
              tunnel: w623 -> [w629]
              frame #0 {
                n243 = Wait (ms)(milliseconds to wait=u32 100) -> ()  [unwired: 1 out]
              }
            }
          }
          frame True {
            n244 = call "Sigma_TriggerOff.vi"("error in (no error)"=w632, "VISA resource name"=w633) -> ("error out"=w634:errorcluster, "VISA resource name out"=w635:refnum<visa-resource-name>)  [unwired: 8 in]
            n245 = local write "Scan"(FALSE ("Move X")) -> ()
          }
        }
      }
      frame "Wait to destinatioin Y" {
        n246 = local read "Cur. Pos X"() -> (w647:dbl)
        n247 = local read "Cur. Pos Y"() -> (w646:dbl)
        n248 = local read "Travel per Pulse (mm)"() -> (w648:dbl)
        n249 = call "Sigma_GetPos.vi"("VISA resource name"=w644, "Travel per Pulse (mm)"=w648, "Init Pos X (mm)"=w647, "Init  Pos Y (mm)"=w646, "error in (no error)"=w643) -> ("Pos X (mm)"=w645:dbl, "Pos Y (mm)"=w637:dbl, "VISA resource name out"=w642:refnum<visa-resource-name>, "error out"=w641:errorcluster)  [unwired: 6 in, 1 out]
        n250 = Absolute Value(x=w651) -> (abs(x)=w657:dbl)
        n251 = Subtract(x=w637, y=w638) -> (x-y=w659:dbl)
        n252 = local write "Cur. Pos X"(w645) -> ()
        n253 = local write "Cur. Pos Y"(w637) -> ()
        n254 = Absolute Value(x=w659) -> (abs(x)=w658:dbl)
        n255 = Subtract(x=w658, y=w657) -> (x-y=w640:dbl)
        n256 = call "Convert Double Precision.vi"("Input"=w640) -> ("Output"=w639:dbl)  [unwired: 10 in]
        n257 = Greater Or Equal To 0?(x=w639) -> (x >= 0?=w654:bool)
        n258 = case shown="False" w654 {
          tunnel: [T3."Wait to destinatioin Y" T3."Move X"] -> w653
          tunnel: w638 -> [w662 _]
          tunnel: [w662 w669] -> w652
          tunnel: [w661 w668] -> w650
          tunnel: [w660 w667] -> w649
          tunnel: w642 -> [w661 w668]
          tunnel: w641 -> [w660 w667]
          frame False {
            n259 = disable-structure shown="비활성화" {
              frame Disabled {
                n260 = Wait (ms)(milliseconds to wait=u32 100) -> ()  [unwired: 1 out]
              }
              frame Enabled {
              }
            }
          }
          frame True {
            n261 = local read "Cur. Pos Y"() -> (w669:dbl)
            n262 = local read "Direction (+)"() -> (w666:bool)
            n263 = local write "Move X"(TRUE ("Move X")) -> ()
            n264 = Not(x=w666) -> (.not. x?=w665:bool)
            n265 = local write "Direction (+)"(w665) -> ()
          }
        }
      }
    }
    n266 = Unbundle By Name(w490) -> ("status"=w489:bool)
    n267 = local read "Stop Scan"() -> (w491:bool)
    n268 = Compound Arithmetic op=OR(w489, w491) -> (w488:bool)
  }
  n269 = while {
    shift-right: [w674] -> _
    shift-left: w108 -> [w679]
    shift-right: [w676] -> _
    shift-left: w109 -> [w678]
    stop <- w675 stop-if-true
    n270 = event shown="[0] Timeout" {
      selector: _ -> [_ _ _ _ _ _ _ _ _ _ _]
      dyn-events: _ -> [_ _ _ _ _ _ _ _ _ _ _]
      timeout: 100 -> [_ _ _ _ _ _ _ _ _ _ _]
      tunnel: w679 -> [w684 w717 w730 w733 w748 w763 w778 w795 w807 w817 w829]
      tunnel: w678 -> [w683 w716 w727 w732 w747 w762 w777 w794 w806 w816 w828]
      tunnel: [w682 w717 w729 w735 w750 w765 w780 w792 w805 w819 w831] -> w674
      tunnel: [w681 w716 w728 w734 w749 w764 w779 w791 w804 w818 w830] -> w676
      tunnel: [_ "Stop Scan" _ _ _ _ _ _ _ _ _] -> w673
      event Timeout {
        n271 = event-data() -> ()  [unwired: 1 in, 2 out]
        n272 = local read "Scan"() -> (w680:bool)
        n273 = case shown="False" w680 {
          tunnel: w684 -> [w696 w715]
          tunnel: w683 -> [w695 w714]
          tunnel: [w694 w715] -> w682
          tunnel: [w693 w714] -> w681
          frame False {
            # "Stop at LS"
            n274 = local read "Cur. Pos X"() -> (w686:dbl)
            n275 = local read "Cur. Pos Y"() -> (w685:dbl)
            n276 = local read "Travel per Pulse (mm)"() -> (w688:dbl)
            n277 = call "Sigma_GetPos.vi"("VISA resource name"=w696, "Travel per Pulse (mm)"=w688, "Init Pos X (mm)"=w686, "Init  Pos Y (mm)"=w685, "error in (no error)"=w695) -> ("Pos X (mm)"=w691:dbl, "Pos Y (mm)"=w692:dbl, "VISA resource name out"=w689:refnum<visa-resource-name>, "State String"=w687:string, "error out"=w690:errorcluster)  [unwired: 6 in]
            n278 = local write "Cur. Pos X"(w691) -> ()
            n279 = local write "Cur. Pos Y"(w692) -> ()
            n280 = case shown="\"W\"" w687 {
              tunnel: [w698 w703 w708 w713] -> w694
              tunnel: [w697 w702 w707 w712] -> w693
              tunnel: w689 -> [w698 w700 w705 w710]
              tunnel: w690 -> [w697 w699 w704 w709]
              frame "K", Default {
              }
              frame "L" {
                n281 = call "Sigma_Stop.vi"("Axis (1)"="1", "error in (no error)"=w699, "VISA resource name"=w700) -> ("error out"=w702:errorcluster, "VISA resource name out"=w703:refnum<visa-resource-name>)  [unwired: 7 in]
              }
              frame "M" {
                n282 = call "Sigma_Stop.vi"("Axis (1)"="2", "error in (no error)"=w704, "VISA resource name"=w705) -> ("error out"=w707:errorcluster, "VISA resource name out"=w708:refnum<visa-resource-name>)  [unwired: 7 in]
              }
              frame "W" {
                n283 = call "Sigma_Stop.vi"("Axis (1)"="W", "error in (no error)"=w709, "VISA resource name"=w710) -> ("error out"=w712:errorcluster, "VISA resource name out"=w713:refnum<visa-resource-name>)  [unwired: 7 in]
              }
            }
          }
          frame True {
          }
        }
      }
      event "Stop Scan": Value Change {
        n284 = event-data() -> ()  [unwired: 1 in, 2 out]
      }
      event "Save Speed": Value Change {
        n285 = event-data() -> ()  [unwired: 1 in, 5 out]
        n286 = local read "Travel per Pulse (mm)"() -> (w719:dbl)
        n287 = local read "1  Max"() -> (w724:dbl)
        n288 = local read "1 Rate"() -> (w723:dbl)
        n289 = local read "2 Rate"() -> (w720:dbl)
        n290 = local read "2 Max"() -> (w721:dbl)
        n291 = local read "1 Min"() -> (w725:dbl)
        n292 = local read "2 Min"() -> (w722:dbl)
        n293 = call "Sigma_SetSpeed.vi"("VISA resource name"=w730, "Travel per Pulse (0.004mm)"=w719, "Min (1mm) 2"=w722, "Max (2mm) 2"=w721, "Rate (1mm) 2"=w720, "error in (no error)"=w727, "Axis (1)"="W", "Min (1mm)"=w725, "Max (2mm)"=w724, "Rate (1mm)"=w723) -> ("VISA resource name out"=w729:refnum<visa-resource-name>, "error out"=w728:errorcluster)  [unwired: 8 in]
      }
      event "Right": Value Change {
        n294 = event-data() -> ()  [unwired: 1 in, 1 out]
        n295 = case shown="True" "Right" {
          tunnel: [w737 w743] -> w735
          tunnel: [w736 w742] -> w734
          tunnel: w733 -> [w737 w745]
          tunnel: w732 -> [w736 w744]
          frame False {
          }
          frame True {
            n296 = local read "Travel per Pulse (mm)"() -> (w739:dbl)
            n297 = local read "Move Distance"() -> (w738:dbl)
            n298 = call "Sigma_MoveAbs.vi"("Direction (+)"=FALSE, "Axis (1)"=1, "error in (no error)"=w744, "Travel (1mm)"=w738, "Travel per Pulse (0.004mm)"=w739, "VISA resource name"=w745) -> ("error out"=w742:errorcluster, "VISA resource name out"=w743:refnum<visa-resource-name>)  [unwired: 4 in]
          }
        }
      }
      event "Left": Value Change {
        n299 = event-data() -> ()  [unwired: 1 in, 1 out]
        n300 = case shown="True" "Left" {
          tunnel: [w752 w759] -> w750
          tunnel: [w751 w758] -> w749
          tunnel: w748 -> [w752 w760]
          tunnel: w747 -> [w751 w757]
          frame False {
          }
          frame True {
            n301 = local read "Travel per Pulse (mm)"() -> (w754:dbl)
            n302 = local read "Move Distance"() -> (w753:dbl)
            n303 = call "Sigma_MoveAbs.vi"("Direction (+)"=TRUE, "Axis (1)"=1, "error in (no error)"=w757, "Travel (1mm)"=w753, "Travel per Pulse (0.004mm)"=w754, "VISA resource name"=w760) -> ("error out"=w758:errorcluster, "VISA resource name out"=w759:refnum<visa-resource-name>)  [unwired: 4 in]
          }
        }
      }
      event "Front": Value Change {
        n304 = event-data() -> ()  [unwired: 1 in, 1 out]
        n305 = case shown="True" "Front" {
          tunnel: [w767 w773] -> w765
          tunnel: [w766 w772] -> w764
          tunnel: w763 -> [w767 w775]
          tunnel: w762 -> [w766 w774]
          frame False {
          }
          frame True {
            n306 = local read "Travel per Pulse (mm)"() -> (w769:dbl)
            n307 = local read "Move Distance"() -> (w768:dbl)
            n308 = call "Sigma_MoveAbs.vi"("Direction (+)"=FALSE, "Axis (1)"=2, "error in (no error)"=w774, "Travel (1mm)"=w768, "Travel per Pulse (0.004mm)"=w769, "VISA resource name"=w775) -> ("error out"=w772:errorcluster, "VISA resource name out"=w773:refnum<visa-resource-name>)  [unwired: 4 in]
          }
        }
      }
      event "Back": Value Change {
        n309 = event-data() -> ()  [unwired: 1 in, 1 out]
        n310 = case shown="True" "Back" {
          tunnel: [w782 w788] -> w780
          tunnel: [w781 w787] -> w779
          tunnel: w778 -> [w782 w790]
          tunnel: w777 -> [w781 w789]
          frame False {
          }
          frame True {
            n311 = local read "Travel per Pulse (mm)"() -> (w784:dbl)
            n312 = local read "Move Distance"() -> (w783:dbl)
            n313 = call "Sigma_MoveAbs.vi"("Direction (+)"=TRUE, "Axis (1)"=2, "error in (no error)"=w789, "Travel (1mm)"=w783, "Travel per Pulse (0.004mm)"=w784, "VISA resource name"=w790) -> ("error out"=w787:errorcluster, "VISA resource name out"=w788:refnum<visa-resource-name>)  [unwired: 4 in]
          }
        }
      }
      event "Home X": Value Change {
        n314 = event-data() -> ()  [unwired: 1 in, 1 out]
        n315 = case shown="True" "Home X" {
          tunnel: [w797 w800] -> w792
          tunnel: [w796 w799] -> w791
          tunnel: w795 -> [w797 w802]
          tunnel: w794 -> [w796 w801]
          frame False {
          }
          frame True {
            n316 = call "Sigma_Home.vi"("Axis (1)"="1", "error in (no error)"=w801, "VISA resource name"=w802) -> ("error out"=w799:errorcluster, "VISA resource name out"=w800:refnum<visa-resource-name>)  [unwired: 7 in]
          }
        }
      }
      event "Home Y": Value Change {
        n317 = event-data() -> ()  [unwired: 1 in, 1 out]
        n318 = case shown="True" "Home Y" {
          tunnel: [w809 w812] -> w805
          tunnel: [w808 w811] -> w804
          tunnel: w807 -> [w809 w814]
          tunnel: w806 -> [w808 w813]
          frame False {
          }
          frame True {
            n319 = call "Sigma_Home.vi"("Axis (1)"="2", "error in (no error)"=w813, "VISA resource name"=w814) -> ("error out"=w811:errorcluster, "VISA resource name out"=w812:refnum<visa-resource-name>)  [unwired: 7 in]
          }
        }
      }
      event "Stop 3": Value Change {
        n320 = event-data() -> ()  [unwired: 1 in, 1 out]
        n321 = case shown="True" "Stop 3" {
          tunnel: [w821 w822] -> w819
          tunnel: [w820 w823] -> w818
          tunnel: w817 -> [w821 w825]
          tunnel: w816 -> [w820 w824]
          frame False {
          }
          frame True {
            n322 = call "Sigma_Stop.vi"("Axis (1)"="W", "error in (no error)"=w824, "VISA resource name"=w825) -> ("error out"=w823:errorcluster, "VISA resource name out"=w822:refnum<visa-resource-name>)  [unwired: 7 in]
          }
        }
      }
      event "Emergency Stop": Value Change {
        n323 = event-data() -> ()  [unwired: 1 in, 1 out]
        n324 = case shown="True" "Emergency Stop" {
          tunnel: [w833 w836] -> w831
          tunnel: [w832 w835] -> w830
          tunnel: w829 -> [w833 w838]
          tunnel: w828 -> [w832 w837]
          frame False {
          }
          frame True {
            n325 = call "Sigma_Stop.vi"("Axis (1)"="E", "error in (no error)"=w837, "VISA resource name"=w838) -> ("error out"=w835:errorcluster, "VISA resource name out"=w836:refnum<visa-resource-name>)  [unwired: 7 in]
          }
        }
      }
    }
    n326 = Unbundle By Name(w676) -> ("status"=w677:bool)
    n327 = Compound Arithmetic op=OR(w677, w673) -> (w675:bool)
  }
  n328 = call <vilib>:"DAQmx Start Task.vi"("task/channels in"=w13, "error in"=w14) -> ("task out"=w15:refnum<k21>, "error out"=w12:errorcluster)  [unwired: 12 in]
  n329 = while {
    tunnel: w15 -> [w849]
    tunnel: w12 -> [w848]
    tunnel: [w841] -> w11
    tunnel: [w847] -> w21
    tunnel: [w840] -> _
    tunnel: w10 -> [w840]
    stop <- w842 stop-if-true
    n330 = call-poly <vilib>:"DAQmx Read.vi"("task/channels in"=w849, "error in"=w848) -> ("task out"=w847:refnum<k21>, "data"=→"Motor Pulse Count":u32, "error out"=w841:errorcluster)  [unwired: 11 in]
    n331 = Wait Until Next ms Multiple(millisecond multiple=u32 10 ("milliseconds to wait")) -> ()  [unwired: 1 out]
    n332 = local read "Completed"() -> (w843:bool)
    n333 = Unbundle By Name(w841) -> ("status"=w845:bool)
    n334 = local read "Stop Scan"() -> (w844:bool)
    n335 = Compound Arithmetic op=OR(w845, w843, w844) -> (w842:bool)
  }
  n336 = call <vilib>:"DAQmx Stop Task.vi"("task/channels in"=w21, "error in"=w11) -> ("task out"=w23:refnum<k21>, "error out"=w22:errorcluster)  [unwired: 12 in]
  n337 = call <vilib>:"Simple Error Handler.vi"("error in (no error)"=w11) -> ()  [unwired: 4 in, 5 out]
  n338 = call <vilib>:"DAQmx Clear Task.vi"("task in"=w23, "error in"=w22) -> ("error out"=w16:errorcluster)  [unwired: 13 in]
  n339 = call <vilib>:"Simple Error Handler.vi"("error in (no error)"=w16) -> ()  [unwired: 4 in, 5 out]
  n340 = VISA Close(VISA resource name=w52, error in (no error)=w53) -> (error out=w51:errorcluster)
  n341 = call <vilib>:"Simple Error Handler.vi"("error in (no error)"=w51) -> ()  [unwired: 4 in, 5 out]
  n342 = call <vilib>:"DAQmx Clear Task.vi"("task in"=w75, "error in"=w74) -> ("error out"=w80:errorcluster)  [unwired: 13 in]
  n343 = call <vilib>:"Simple Error Handler.vi"("error in (no error)"=w80) -> ()  [unwired: 4 in, 5 out]
  n344 = call <vilib>:"Simple Error Handler.vi"() -> ()  [unwired: 5 in, 5 out]
  "Move X" <- FALSE ("Move X")
